vi "item select invert calc.vi"(7 "Action":T1, 9 "selection index":i32, 10 "selection locks":bool[](array[boolean]), 11 "selection states":bool[](array[boolean])) -> (3 "new selection states":bool[](array[boolean]))   [LabVIEW 2020, in "UI_ItemSelect.lvlib"]
uses:
  UI_ItemSelect.lvlib
  item select calc action.ctl
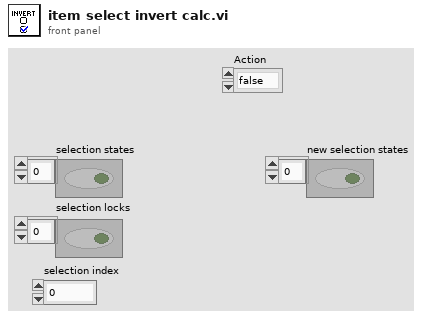
[diagram p1: front panel]
types:
  T1 = typedef "UI_ItemSelect.lvlib/item select calc action.ctl" = enum16{"false", "true", "invert"}
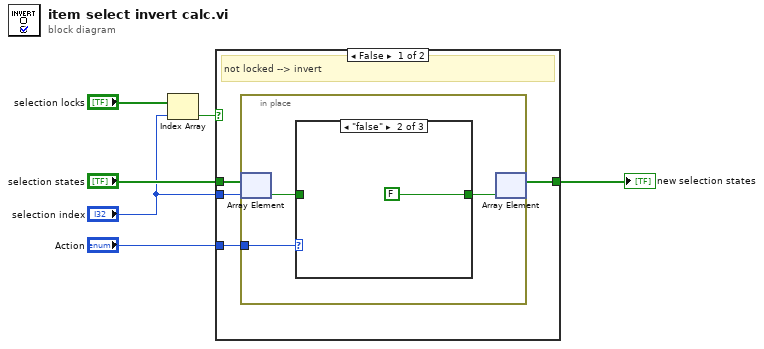
[diagram p0: block diagram]
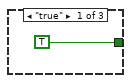
[diagram p2: hidden frame]
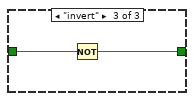
[diagram p3: hidden frame]
diagram:
  n1 = Index Array(array="selection locks", index="selection index") -> (element=w3:bool)
  n2 = case shown="False" w3 {
    tunnel: "selection states" -> [w10 w18]
    tunnel: [w9 w18] -> w4
    tunnel: "selection index" -> [w8 _]
    tunnel: "Action" -> [w7 _]
    frame False {
      # "not locked --> invert"
      n3 = in-place {
        in-place-border: w7 -> [w11]
        n4 = in-place-array #1(w10, w8) -> (w13:bool)
        n5 = case shown="\"false\"" w11 {
          tunnel: w13 -> [_ _ w17]
          tunnel: [TRUE FALSE w16] -> w12
          frame "true" {
          }
          frame "false" {
          }
          frame "invert" {
            n6 = Not(x=w17) -> (.not. x?=w16:bool)
          }
        }
        n7 = in-place-array #1(w12) -> (w9:bool[])  [unwired: 1 out]
      }
    }
    frame True {
      # "locked!  don't touch"
    }
  }
  "new selection states" <- w4
